vi "NicmosSetDIO.vi"(9 "error in (no error)":errorcluster caption="entrée d'erreur") -> (0 "NICMOS task out":refnum<k21>, 6 "error out":errorcluster caption="sortie d'erreur")   [LabVIEW 2009]
uses:
  <vilib>/DAQmx/configure/trigger.llb/DAQmx Start Trigger (Digital Edge).vi
  <vilib>/DAQmx/configure/timing.llb/DAQmx Timing (Sample Clock).vi
  <vilib>/DAQmx/create/channels.llb/DAQmx Create Channel (DI-Digital Input).vi
  <vilib>/DAQmx/configure/events/hardwareSignals.llb/DAQmx Export Signal (Most Signals).vi
panel:
  in  "Case Constant\n(See Context Help)":bool=TRUE
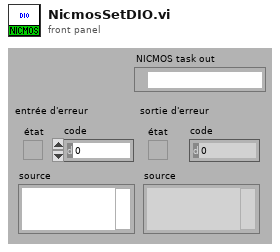
[diagram p1: front panel]
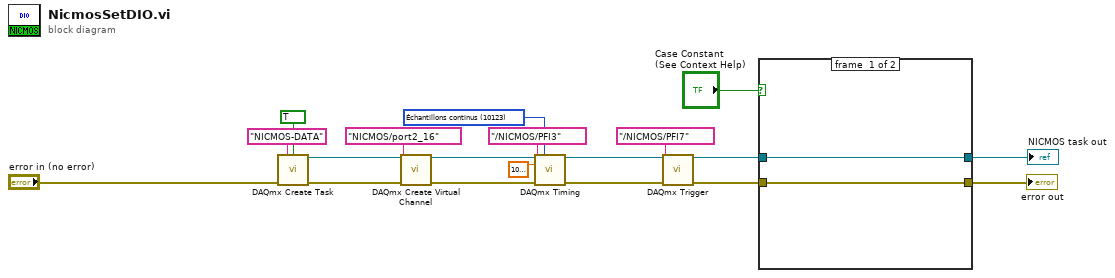
[diagram p0: block diagram]
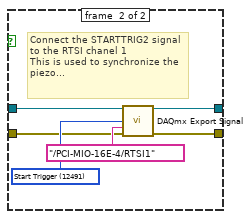
[diagram p2: hidden frame]
diagram:
  w4 = 10123 items=["Échantillons finis"=10178, "Échantillons continus"=10123, "Point par point avec cadencement matériel"=12522] ("sample mode")
  n1 = call <vilib>:"DAQmx Create Task.vi"("new task name"="NICMOS-DATA", "auto cleanup"=TRUE, "error in"="error in (no error)") -> ("task out"=w15:refnum<k21>, "error out"=w16:errorcluster)  [unwired: 11 in]
  n2 = call-poly <vilib>:"DAQmx Create Virtual Channel.vi"("task in"=w15, "lines"=tag "NICMOS/port2_16", "error in"=w16) -> ("task out"=w12:refnum<k21>, "error out"=w13:errorcluster)  [unwired: 11 in]
  n3 = call-poly <vilib>:"DAQmx Timing.vi"("task/channels in"=w12, "sample mode"=w4, "rate"=1000000.0, "source"=tag "/NICMOS/PFI3", "error in"=w13) -> ("task out"=w8:refnum<k21>, "error out"=w9:errorcluster)  [unwired: 9 in]
  n4 = call-poly <vilib>:"DAQmx Trigger.vi"("task/channels in"=w8, "source"=tag "/NICMOS/PFI7", "error in"=w9) -> ("task out"=w5:refnum<k21>, "error out"=w6:errorcluster)  [unwired: 11 in]
  n5 = case shown="True" "Case Constant\n(See Context Help)" {
    tunnel: [w20 w27] -> w19
    tunnel: [w21 w26] -> w18
    tunnel: w6 -> [w20 w23]
    tunnel: w5 -> [w21 w22]
    frame #0 {
    }
    frame #1 {
      w25 = 12491 items=["AI Convert Clock"=12484, "10MHz Reference Clock"=12536, "20MHz Timebase Clock"=12486, "Sample Clock"=12487, "Déclenchement d'avancement"=12488, "Reference Trigger"=12490, "Start Trigger"=12491, "Advance Complete Event"=12492, "AI Hold Complete Event"=12493, "Counter Output Event"=12494, "Change Detection Event"=12511, "Watchdog Timer Expired Event"=12512] ("signal")
      # "Connect the STARTTRIG2 signal to the RTSI chanel 1\nThis is used to synchronize the piezo..."
      n6 = call-poly <vilib>:"DAQmx Export Signal.vi"("task/channels in"=w22, "signal"=w25, "output terminal"=tag "/PCI-MIO-16E-4/RTSI1", "error in"=w23) -> ("task out"=w26:refnum<k21>, "error out"=w27:errorcluster)  [unwired: 10 in]
    }
  }
  "error out" <- w19
  "NICMOS task out" <- w18
